vi "Read Filter.vi"(8 "error in (no error)":errorcluster, 11 "ElectrometerInternalConfiguration in":refnum<class "ElectrometerInternalConfiguration.lvclass">) -> (0 "error out":errorcluster, 2 "Filter":T1, 3 "ElectrometerInternalConfiguration out":refnum<class "ElectrometerInternalConfiguration.lvclass">)   [LabVIEW 2016, in "ElectrometerInternalConfiguration.lvclass"]
uses:
  ElectrometerInternalConfiguration.lvclass
  Electrometer/MED Filter Type.ctl
  ElectrometerInternalConfiguration.lvclass/ElectrometerInternalConfiguration.ctl
  Electrometer/Electrometer.lvclass
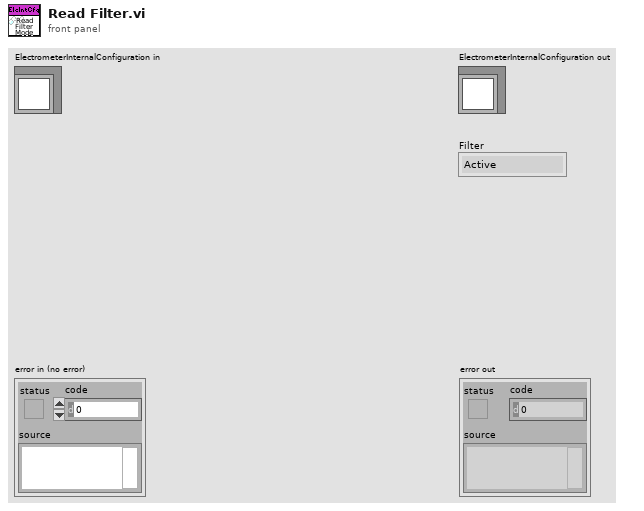
[diagram p1: front panel]
types:
  T1 = typedef "Electrometer.lvclass/MED Filter Type.ctl" = enum16{"Active", "None"}
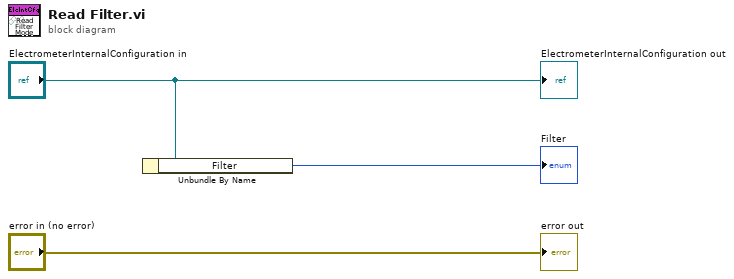
[diagram p0: block diagram]
diagram:
  n1 = Unbundle By Name("ElectrometerInternalConfiguration in") -> ("Filter"=→"Filter":T1)
  "error out" <- "error in (no error)"
  "ElectrometerInternalConfiguration out" <- "ElectrometerInternalConfiguration in"
